vi "Main.vi"() -> ()   [LabVIEW 2013]
uses:
  <vilib>/myRIO/Instrument Drivers/Onboard IO/SPI/typedefs/SPI User Configuration.ctl
  <vilib>/myRIO/Common/Instrument Driver Framework/myRIO v1.0/SPI/typedefs/SPI Clock Phase.ctl
  <vilib>/myRIO/Common/Instrument Driver Framework/myRIO v1.0/SPI/typedefs/SPI Clock Polarity.ctl
  <vilib>/myRIO/Common/Instrument Driver Framework/myRIO v1.0/SPI/typedefs/SPI Data Direction.ctl
  <vilib>/myRIO/Common/Instrument Driver Framework/myRIO v1.0/SPI/typedefs/SPI Frame Length.ctl
  <vilib>/myRIO/Common/Instrument Driver Framework/myRIO v1.0/DIO/vis/myRIO v1.1 Open DIO.vi
  <vilib>/myRIO/Common/Instrument Driver Framework/myRIO v1.0/SPI/vis/myRIO v1.1 Open SPI.vi
  <vilib>/myRIO/Instrument Drivers/Onboard IO/SPI/vis/Write Read.vi
  <vilib>/myRIO/Common/Instrument Driver Framework/myRIO v1.0/UART/vis/myRIO v1.0 Close UART.vi
  <vilib>/myRIO/Common/Instrument Driver Framework/Utilities/vis/Validate Channels.vi
  <vilib>/myRIO/Common/Instrument Driver Framework/myRIO v1.0/DIO/vis/myRIO v1.0 Reserve DIO.vi
  <vilib>/myRIO/Common/Instrument Driver Framework/myRIO v1.0/SPI/vis/myRIO v1.0 Reserve SPI.vi
  <vilib>/myRIO/Common/Instrument Driver Framework/myRIO v1.0/Resource Manager/vis/myRIO v1.0 Reserve Channel List.vi
  <vilib>/myRIO/Common/Instrument Driver Framework/myRIO v1.0/DIO/vis/myRIO v1.0 Build MUX Configuration DIO.vi
  <vilib>/myRIO/Common/Instrument Driver Framework/myRIO v1.0/SPI/vis/myRIO v1.0 Build MUX Configuration SPI.vi
  <vilib>/myRIO/Common/Instrument Driver Framework/myRIO v1.0/Resource Manager/vis/myRIO v1.0 Reserve Channel.vi
  <vilib>/myRIO/Common/Instrument Driver Framework/myRIO v1.0/Resource Manager/vis/myRIO v1.0 Unreserve Channel.vi
  <vilib>/myRIO/Common/Instrument Driver Framework/myRIO v1.0/Resource Manager/vis/myRIO v1.0 Create Configuration List.vi
  <vilib>/myRIO/Common/Instrument Driver Framework/myRIO v1.0/Resource Manager/vis/myRIO v1.0 Build Mutex Name.vi
  <vilib>/myRIO/Common/Instrument Driver Framework/myRIO v1.0/myRIO v1.1 Open.vi
  <vilib>/Utility/VariantDataType/GetNumericInfo.vi
  <vilib>/Utility/error.llb/Error Cluster From Error Code.vi
  <vilib>/myRIO/Common/Instrument Driver Framework/Utilities/vis/IO Manager.vi
  <vilib>/myRIO/Common/Instrument Driver Framework/Utilities/vis/Configuration Manager.vi
  <vilib>/myRIO/Common/Instrument Driver Framework/myRIO v1.0/Resource Manager/vis/myRIO v1.0 Configure IO.vi
  <vilib>/myRIO/Common/Instrument Driver Framework/myRIO v1.0/myRIO v1.0 Close.vi
  <vilib>/myRIO/Common/Instrument Driver Framework/myRIO v1.0/SPI/vis/myRIO v1.0 Configure SPI.vi
  <vilib>/myRIO/Common/Instrument Driver Framework/myRIO v1.0/DIO/vis/myRIO v1.0 Write DIO.vi
  <vilib>/myRIO/Common/Instrument Driver Framework/myRIO v1.0/SPI/vis/myRIO v1.0 Write Read SPI.vi
  <vilib>/myRIO/Common/Instrument Driver Framework/Utilities/vis/FPGA Ref Manager.vi
  <vilib>/myRIO/Common/Instrument Driver Framework/myRIO v1.0/myRIO v1.0 Reset FPGA.vi
  <vilib>/myRIO/Instrument Drivers/Onboard IO/SPI/SPI.lvlib
  <vilib>/myRIO/Instrument Drivers/Onboard IO/DIO/DIO.lvlib
  <vilib>/myRIO/Instrument Drivers/Utilities/Utilities.lvlib
panel:
  in  "ESC":bool
  out "STATUS after read":u16[](array[numeric]) format="%02x"
  out "EEPROM array":u16[](array[numeric]) format="%0d"
  in  "Write protect":bool=TRUE
  in  "Bytes to write":u16[](array[numeric])=[0] max=255 step=1 format="%0d"
  in  "Starting address":u16 max=511 step=1 format="%0d"
  in  "STATUS to write":u16 format="%02x"
  in  "Action":T1(ring)
  out "EEPROM array (graph)":u16[](graph)
  # "EEPROM demo"
  # "Data read from array:"
  # "Data to write to array:"
  # "STATUS byte:"
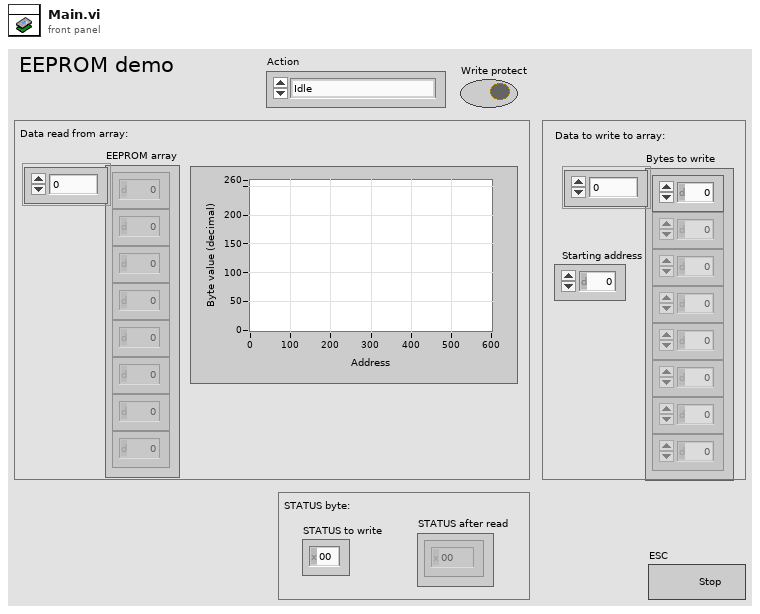
[diagram p1: front panel]
types:
  T1 = enum16{"Idle", "Read entire array", "Write to array", "Read STATUS register", "Write STATUS register"}
  T2 = typedef "SPI.lvlib/SPI User Configuration.ctl" = cluster{"Frequency (Hz)":dbl, "Clock Phase":T3, "Clock Polarity":T4, "Data Direction":T5, "Frame Length":T6}
  T3 = typedef "SPI Clock Phase.ctl" = enum8{"Leading", "Trailing"}
  T4 = typedef "SPI Clock Polarity.ctl" = enum8{"Low", "High"}
  T5 = typedef "SPI Data Direction.ctl" = enum8{"Most Significant Bit First", "Least Significant Bit First"}
  T6 = typedef "SPI Frame Length.ctl" = u8
  T7 = typedef "DIO.lvlib/DIO Reference.ctl" = cluster{"myRIO Reference":T8, "DIO Channels List":T12}
  T8 = typedef "myRIO Generic Hardware Reference.ctl" = cluster{"myRIO Model":T9, "myRIO Hardware Reference":T10}
  T9 = typedef "Hardware Version Enum.ctl" = enum16{"Unknown", "myRIO-1900", "myRIO-1950"}
  T10 = typedef "myRIO v1.0 Reference.ctl" = cluster{"Generic FPGA Reference":T11, "Allow multiple opens":bool}
  T11 = typedef "Generic FPGA Reference.ctl" = refnum<k20>
  T12 = typedef "DIO Channels List.ctl" = T13[]
  T13 = typedef "DIO Channels Enum.ctl" = enum16{"Not Connected", "C/DIO0", "C/DIO1", "C/DIO2", "C/DIO3", "C/DIO4", "C/DIO5", "C/DIO6", "C/DIO7", "A/DIO0", "A/DIO1", "A/DIO2", "A/DIO3", "A/DIO4", "A/DIO5", "A/DIO6", "A/DIO7", "A/DIO8", "A/DIO9", "A/DIO10", "A/DIO11", "A/DIO12", "A/DIO13", "A/DIO14", "A/DIO15", "B/DIO0", "B/DIO1", "B/DIO2", "B/DIO3", "B/DIO4", "B/DIO5", "B/DIO6", "B/DIO7", "B/DIO8", "B/DIO9", "B/DIO10", "B/DIO11", "B/DIO12", "B/DIO13", "B/DIO14", "B/DIO15", "LED0", "LED1", "LED2", "LED3", "Button0"}
  T14 = typedef "SPI.lvlib/SPI Reference.ctl" = cluster{"myRIO Reference":T8, "SPI Channels Enum":T15, "SPI Configuration":T16}
  T15 = typedef "SPI Channels Enum.ctl" = enum16{"Not Connected", "A/SPI", "B/SPI"}
  T16 = typedef "SPI.lvlib/SPI Configuration.ctl" = cluster{"Frequency (Hz)":dbl, "Clock Phase":T3, "Clock Polarity":T4, "Data Direction":T5, "Frame Length":T6}
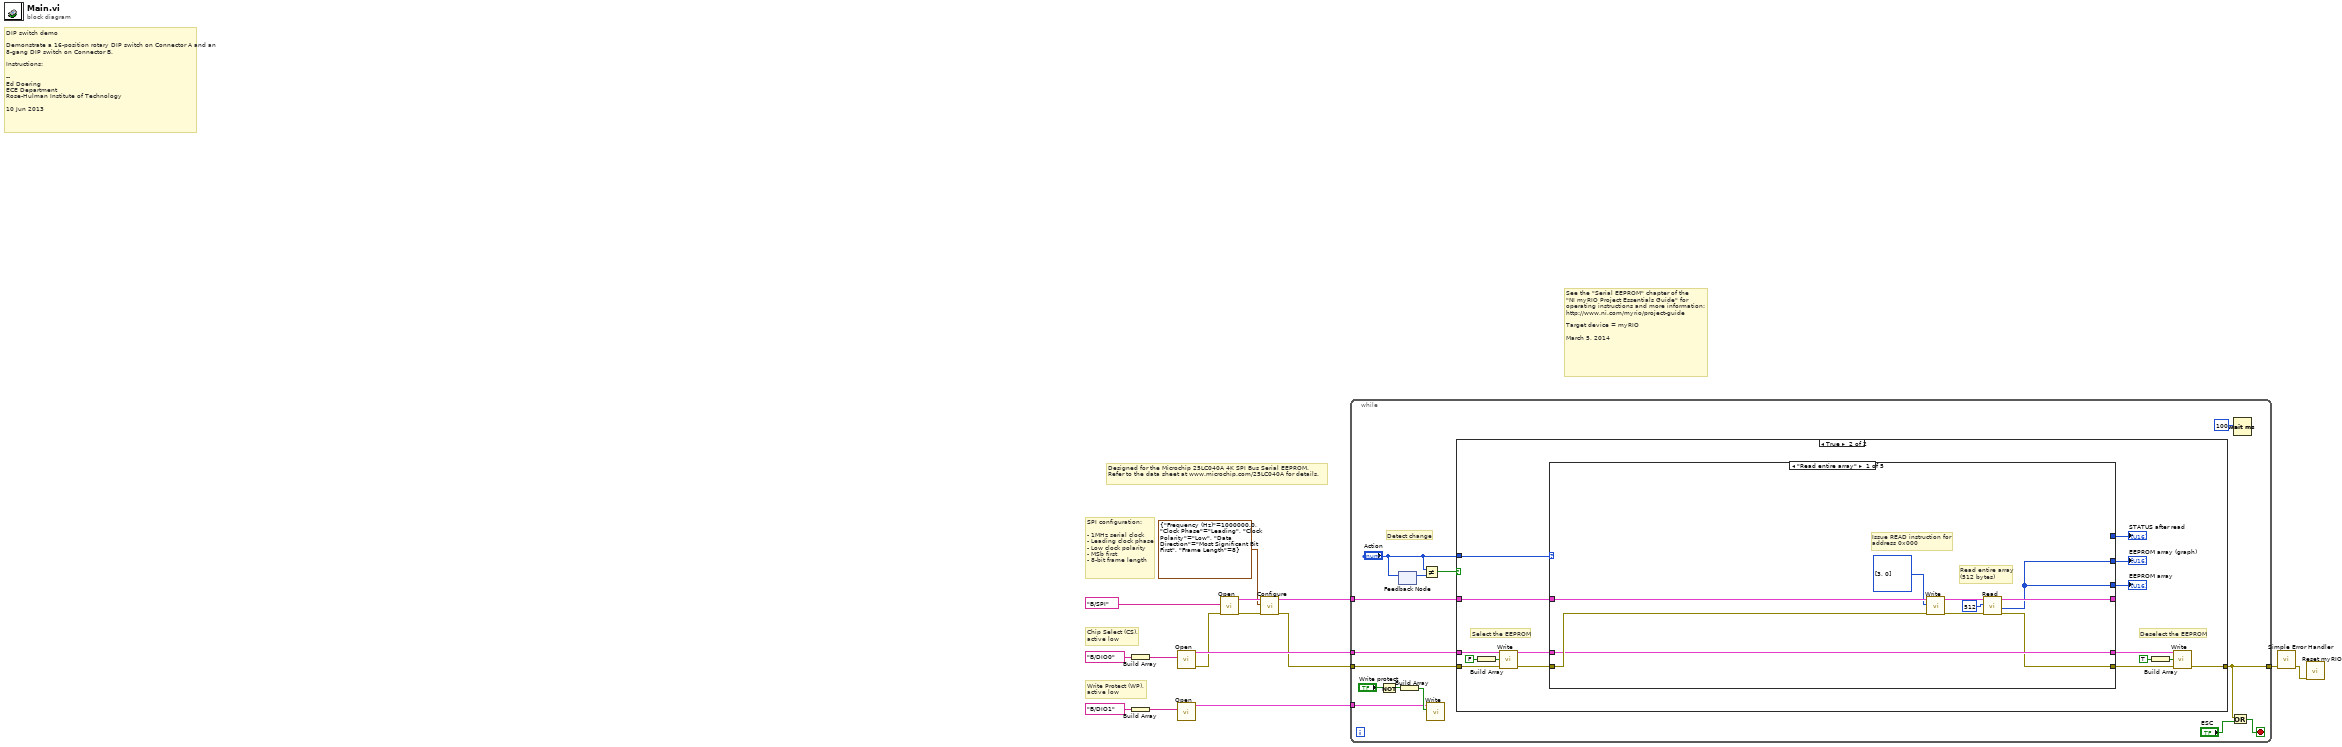
[diagram p0: block diagram]
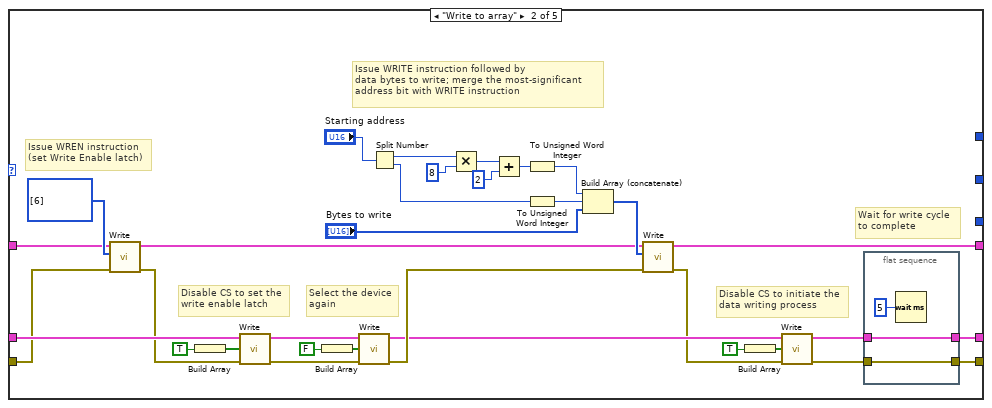
[diagram p3: hidden frame]
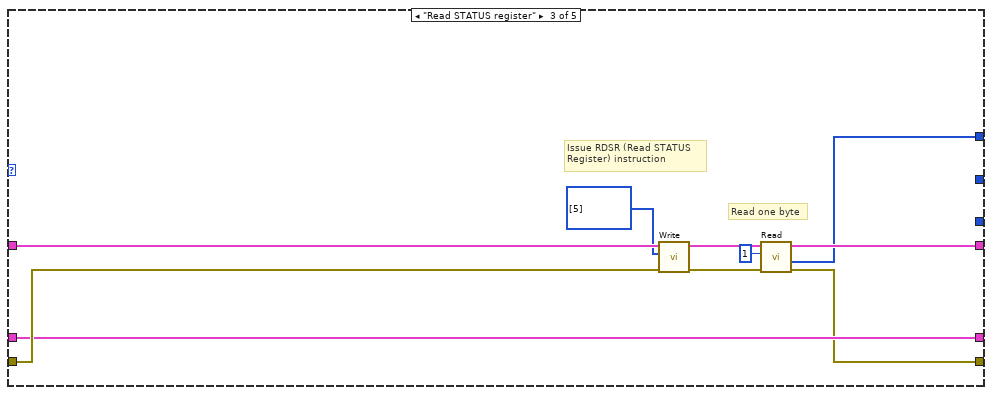
[diagram p4: hidden frame]
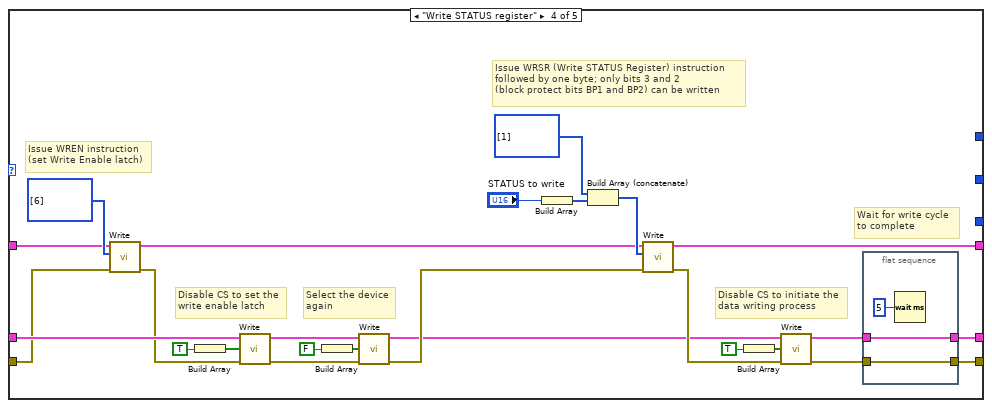
[diagram p5: hidden frame]
diagram:
  # "See the \"Serial EEPROM\" chapter of the\n\"NI myRIO Project Essentials Guide\" for\noperating instructions and more information: \nhttp://www.ni.com/myrio/project-guide\n\nTarget device = myRIO\n\nMarch 5, 2014"
  # "Write Protect (WP),\nactive low"
  # "Chip Select (CS),\nactive low"
  # "SPI configuration:\n\n- 1MHz serial clock\n- Leading clock phase\n- Low clock polarity\n- MSb first\n- 8-bit frame length"
  # "Designed for the Microchip 25LC040A 4K SPI Bus Serial EEPROM.\nRefer to the data sheet at www.microchip.com/25LC040A for details."
  # "DIP switch demo\n\nDemonstrate a 16-position rotary DIP switch on Connector A and an 8-gang DIP switch on Connector B.\n\nInstructions:\n\n-- \nEd Doering\nECE Department\nRose-Hulman Institute of Technology\n\n10 Jun 2013"
  n1 = Build Array "Build Array"(tag "B/DIO0" ("myRIO DIO Channel")) -> (w9:tag[])
  n2 = Build Array(tag "B/DIO1" ("myRIO DIO Channel")) -> (w6:tag[])
  n3 = call <vilib>:"Open.vi"("Channel Names"=w9) -> ("error out"=w10:errorcluster, "DIO Ref Out"=w11:T7)  [unwired: 9 in]
  n4 = call <vilib>:"Open.vi"("Channel Names"=w6) -> ("DIO Ref Out"=w1:T7)  [unwired: 9 in, 1 out]
  n5 = call <vilib>:"Open.vi"("error in (no error)"=w10, "Channel Name"=tag "B/SPI") -> ("error out"=w12:errorcluster, "SPI Ref Out"=w14:T14)  [unwired: 8 in]
  n6 = call <vilib>:"Configure.vi"("error in (no error)"=w12, "SPI User Configuration"=T2 {"Frequency (Hz)"=1000000.0, "Clock Phase"=enum."Leading", "Clock Polarity"=enum."Low", "Data Direction"=enum."Most Significant Bit First", "Frame Length"=8}, "SPI Ref In"=w14) -> ("error out"=w4:errorcluster, "SPI Ref Out"=w13:T14)  [unwired: 7 in]
  n7 = while {
    tunnel: w13 -> [w29]
    tunnel: w11 -> [w28]
    tunnel: w4 -> [w27]
    tunnel: [w19] -> w3
    tunnel: w1 -> [w20]
    stop <- w17 stop-if-true
    # "Detect change"
    n8 = Not(x="Write protect") -> (.not. x?=w23:bool)
    n9 = feedback #1() -> (w24:T1)  [unwired: 1 in]
    n10 = feedback-in #1("Action") -> ()
    n11 = Build Array(w23) -> (w21:bool[])
    n12 = Not Equal?(x="Action", y=w24) -> (x != y?=w26:bool)
    n13 = call <vilib>:"Write.vi"("Values"=w21, "DIO Ref In"=w20) -> ()  [unwired: 7 in, 2 out]
    n14 = case shown="True" w26 {
      tunnel: w29 -> [_ w46]
      tunnel: w28 -> [_ w45]
      tunnel: "Action" -> [_ w37]
      tunnel: w27 -> [w30 w32]
      tunnel: [w30 w31] -> w19
      frame False {
      }
      frame True {
        # "Deselect the EEPROM"
        # "Select the EEPROM"
        n15 = Build Array(FALSE) -> (w43:bool[])
        n16 = call <vilib>:"Write.vi"("error in (no error)"=w32, "Values"=w43, "DIO Ref In"=w45) -> ("error out"=w42:errorcluster, "DIO Ref Out"=w39:T7)  [unwired: 6 in]
        n17 = case shown="\"Read entire array\"" w37 {
          tunnel: w46 -> [w56 w71 w102 w117 w134]
          tunnel: w42 -> [w55 w58 w101 w104 w133]
          tunnel: [w50 w89 w97 w128 w134] -> _
          tunnel: [w48 w59 w95 w107 w133] -> w36
          tunnel: w39 -> [w53 w72 w99 w119 w132]
          tunnel: [w53 w61 w99 w105 w132] -> w38
          tunnel: [w47 _ _ _ _] -> w35
          tunnel: [w47 _ _ _ _] -> w34
          tunnel: [_ _ w93 _ _] -> w33
          frame "Read entire array" {
            # "Read entire array\n(512 bytes)"
            # "Issue READ instruction for\naddress 0x000"
            n18 = call <vilib>:"Write.vi"("error in (no error)"=w55, "Frames to Write"=u16[] [3, 0], "SPI Ref In"=w56) -> ("error out"=w49:errorcluster, "SPI Ref Out"=w51:T14)  [unwired: 7 in]
            n19 = call <vilib>:"Read.vi"("error in (no error)"=w49, "Frame Count"=u32 512, "SPI Ref In"=w51) -> ("error out"=w48:errorcluster, "Frames Read"=w47:u16[], "SPI Ref Out"=w50:T14)  [unwired: 5 in]
          }
          frame "Write to array" {
            # "Wait for write cycle\nto complete"
            # "Disable CS to initiate the\ndata writing process"
            # "Select the device\nagain"
            # "Issue WREN instruction\n(set Write Enable latch)"
            # "Disable CS to set the\nwrite enable latch"
            # "Issue WRITE instruction followed by\ndata bytes to write; merge the most-significant\naddress bit with WRITE instruction"
            n20 = call <vilib>:"Write.vi"("error in (no error)"=w58, "Frames to Write"=u16[] [6], "SPI Ref In"=w71) -> ("error out"=w57:errorcluster, "SPI Ref Out"=w70:T14)  [unwired: 7 in]
            n21 = Build Array(TRUE) -> (w76:bool[])
            n22 = call <vilib>:"Write.vi"("error in (no error)"=w57, "Values"=w76, "DIO Ref In"=w72) -> ("error out"=w75:errorcluster, "DIO Ref Out"=w77:T7)  [unwired: 6 in]
            n23 = Build Array(FALSE) -> (w67:bool[])
            n24 = call <vilib>:"Write.vi"("error in (no error)"=w75, "Values"=w67, "DIO Ref In"=w77) -> ("error out"=w69:errorcluster, "DIO Ref Out"=w64:T7)  [unwired: 6 in]
            n25 = Split Number(x="Starting address") -> (hi(x)=w87:u8, lo(x)=w82:u8)
            n26 = Multiply(x=w87, y=u8 8) -> (x*y=w85:u8)
            n27 = Add(x=w85, y=u8 2) -> (x+y=w83:u8)
            n28 = To Unsigned Word Integer(number=w83) -> (unsigned 16bit integer=w81:u16)
            n29 = To Unsigned Word Integer(number=w82) -> (unsigned 16bit integer=w80:u16)
            n30 = Build Array (concatenate) "Build Array"(w81, w80, "Bytes to write") -> (w78:u16[])
            n31 = call <vilib>:"Write.vi"("error in (no error)"=w69, "Frames to Write"=w78, "SPI Ref In"=w70) -> ("error out"=w63:errorcluster, "SPI Ref Out"=w89:T14)  [unwired: 7 in]
            n32 = Build Array(TRUE) -> (w65:bool[])
            n33 = call <vilib>:"Write.vi"("error in (no error)"=w63, "Values"=w65, "DIO Ref In"=w64) -> ("error out"=w60:errorcluster, "DIO Ref Out"=w62:T7)  [unwired: 6 in]
            n34 = flat-sequence {
              tunnel: w62 -> [w91]
              tunnel: [w91] -> w61
              tunnel: w60 -> [w90]
              tunnel: [w90] -> w59
              frame #0 {
                n35 = Wait (ms)(milliseconds to wait=u32 5) -> ()  [unwired: 1 out]
              }
            }
          }
          frame "Read STATUS register" {
            # "Read one byte"
            # "Issue RDSR (Read STATUS \nRegister) instruction"
            n36 = call <vilib>:"Write.vi"("error in (no error)"=w101, "Frames to Write"=u16[] [5], "SPI Ref In"=w102) -> ("error out"=w96:errorcluster, "SPI Ref Out"=w98:T14)  [unwired: 7 in]
            n37 = call <vilib>:"Read.vi"("error in (no error)"=w96, "Frame Count"=u32 1, "SPI Ref In"=w98) -> ("error out"=w95:errorcluster, "Frames Read"=w93:u16[], "SPI Ref Out"=w97:T14)  [unwired: 5 in]
          }
          frame "Write STATUS register" {
            # "Wait for write cycle\nto complete"
            # "Disable CS to initiate the\ndata writing process"
            # "Issue WREN instruction\n(set Write Enable latch)"
            # "Select the device\nagain"
            # "Disable CS to set the\nwrite enable latch"
            # "Issue WRSR (Write STATUS Register) instruction\nfollowed by one byte; only bits 3 and 2\n(block protect bits BP1 and BP2) can be written"
            n38 = call <vilib>:"Write.vi"("error in (no error)"=w104, "Frames to Write"=u16[] [6], "SPI Ref In"=w117) -> ("error out"=w103:errorcluster, "SPI Ref Out"=w116:T14)  [unwired: 7 in]
            n39 = Build Array(TRUE) -> (w114:bool[])
            n40 = call <vilib>:"Write.vi"("error in (no error)"=w103, "Values"=w114, "DIO Ref In"=w119) -> ("error out"=w115:errorcluster, "DIO Ref Out"=w113:T7)  [unwired: 6 in]
            n41 = Build Array(FALSE) -> (w120:bool[])
            n42 = call <vilib>:"Write.vi"("error in (no error)"=w115, "Values"=w120, "DIO Ref In"=w113) -> ("error out"=w118:errorcluster, "DIO Ref Out"=w109:T7)  [unwired: 6 in]
            n43 = Build Array("STATUS to write") -> (w125:u16[])
            n44 = Build Array (concatenate) "Build Array"(u16[] [1] ("Frames to Write"), w125) -> (w124:u16[])
            n45 = call <vilib>:"Write.vi"("error in (no error)"=w118, "Frames to Write"=w124, "SPI Ref In"=w116) -> ("error out"=w110:errorcluster, "SPI Ref Out"=w128:T14)  [unwired: 7 in]
            n46 = Build Array(TRUE) -> (w111:bool[])
            n47 = call <vilib>:"Write.vi"("error in (no error)"=w110, "Values"=w111, "DIO Ref In"=w109) -> ("error out"=w108:errorcluster, "DIO Ref Out"=w106:T7)  [unwired: 6 in]
            n48 = flat-sequence {
              tunnel: w106 -> [w130]
              tunnel: [w130] -> w105
              tunnel: w108 -> [w129]
              tunnel: [w129] -> w107
              frame #0 {
                n49 = Wait (ms)(milliseconds to wait=u32 5) -> ()  [unwired: 1 out]
              }
            }
          }
          frame "Idle", Default {
          }
        }
        "EEPROM array (graph)" <- w35
        "EEPROM array" <- w34
        "STATUS after read" <- w33
        n50 = Build Array(TRUE) -> (w41:bool[])
        n51 = call <vilib>:"Write.vi"("error in (no error)"=w36, "Values"=w41, "DIO Ref In"=w38) -> ("error out"=w31:errorcluster)  [unwired: 6 in, 1 out]
      }
    }
    n52 = Or(x=w19, y="ESC") -> (x .or. y?=w17:bool)
    n53 = Wait (ms)(milliseconds to wait=u32 100) -> ()  [unwired: 1 out]
  }
  n54 = call <vilib>:"Simple Error Handler.vi"("error in (no error)"=w3) -> ("error out"=w2:errorcluster)  [unwired: 4 in, 4 out]
  n55 = call <vilib>:"Reset myRIO.vi"("error in (no error)"=w2) -> ()  [unwired: 10 in, 1 out]
